vi "Configure RFSG.vi"(0 "Scalar SG Si2250 Path in":refnum<class "SG SC2250 Path.lvclass">, 5 "Cal point in":T1, 7 "External Gain (0 dB)":dbl, 9 "Digital Gain (0 dB)":dbl, 11 "error in (no error)":errorcluster) -> (4 "Scalar SG Si2250 Path out":refnum<class "SG SC2250 Path.lvclass">, 6 "Cal point out":T1, 15 "error out":errorcluster)   [LabVIEW 2023, in "RFFixtureCharact.RFPM.lvlib" / "SG SC2250 Path.lvclass"]
uses:
  SG SC2250 Path.lvclass
  C:/srd-semi-rfcal-software/AuxTools/STSRFFixtureCharactUtility/Source/Code Modules/Fixture/Public/Base Classes/Scalar/Scalar Path/Scalar Path.lvclass
  Public/Base Classes/Scalar/Scalar Path/Type Definitions/Cal Point.ctl
  Public/Base Classes/Scalar/Scalar Path/Scalar Path.lvclass
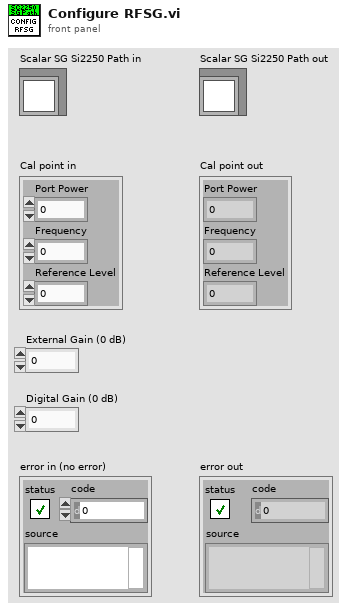
[diagram p1: front panel]
types:
  T1 = typedef "RFFixtureCharact.Public.lvlib/Scalar Path.lvclass/Cal Point.ctl" = cluster{"Port Power":dbl, "Frequency":dbl, "Reference Level":dbl}
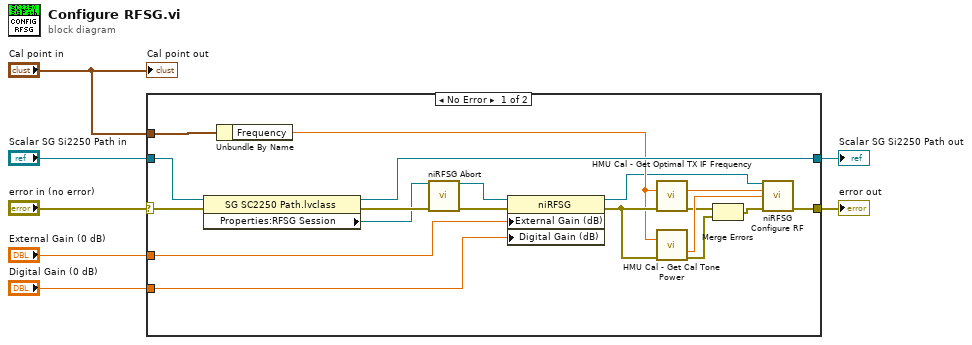
[diagram p0: block diagram]
diagram:
  n1 = case shown="No Error" "error in (no error)" {
    selector: "error in (no error)" -> [w24 w28]
    tunnel: [w25 w28] -> w7
    tunnel: [w21 w27] -> w6
    tunnel: "Scalar SG Si2250 Path in" -> [w22 w27]
    tunnel: "Cal point in" -> [w23 _]
    tunnel: "External Gain (0 dB)" -> [w9 _]
    tunnel: "Digital Gain (0 dB)" -> [w8 _]
    frame No Error {
      n2 = property class="SG SC2250 Path.lvclass"(reference=w22, error in=w24) -> (reference out=w21:refnum<class "SG SC2250 Path.lvclass">, error out=w26:errorcluster, "Properties:RFSG Session"=w17:refnum<k15>)
      n3 = Unbundle By Name(w23) -> ("Frequency"=w14:dbl)
      n4 = call <instrlib>:"niRFSG Abort.vi"("instrument handle"=w17, "error in"=w26) -> ("instrument handle out"=w16:refnum<k15>, "error out"=w18:errorcluster)  [unwired: 12 in]
      n5 = property class="niRFSG"(reference=w16, error in=w18, "External Gain (dB)"=w9, "Digital Gain (dB)"=w8) -> (reference out=w10:refnum<k15>, error out=w15:errorcluster)
      n6 = call "HMU Cal - Get Optimal TX IF Frequency.vi"("RF Frequency (Hz)"=w14, "error in (no error)"=w15) -> ("IF Frequency (Hz)"=w13:dbl, "error out"=w11:errorcluster)  [unwired: 12 in]
      n7 = call "HMU Cal - Get Cal Tone Power.vi"("Tone Frequency (Hz)"=w14, "error in (no error)"=w15) -> ("Coerced RFout Power (dBm)"=w19:dbl, "error out"=w20:errorcluster)  [unwired: 12 in]
      n8 = Merge Errors(w11, w20) -> (w12:errorcluster)
      n9 = call <instrlib>:"niRFSG Configure RF.vi"("instrument handle"=w10, "frequency (Hz)"=w13, "power level (dBm)"=w19, "error in"=w12) -> ("error out"=w25:errorcluster)  [unwired: 10 in, 1 out]
    }
    frame Error {
    }
  }
  "error out" <- w7
  "Scalar SG Si2250 Path out" <- w6
  "Cal point out" <- "Cal point in"
